vi "Get Ball.vi"() -> (0 "Field Relative X":dbl, 1 "Robot Relative Y":dbl, 3 "Robot Relative X":dbl, 4 "Ball Found?":bool)   [LabVIEW 2013]
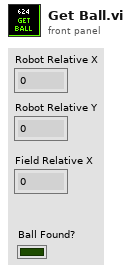
[diagram p1: front panel]
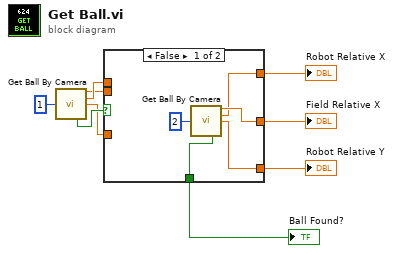
[diagram p0: block diagram]
diagram:
  n1 = call "Get Ball By Camera.vi"("Camera"=i16 1) -> ("Field Relative X"=w3:dbl, "Robot Relative X"=w7:dbl, "Robot Relative Y"=w5:dbl, "Ball Found?"=w8:bool)  [unwired: 9 in, 2 out]
  n2 = case shown="False" w8 {
    selector: w8 -> [_ w15]
    tunnel: w7 -> [_ w18]
    tunnel: [w10 w18] -> w6
    tunnel: w5 -> [_ w17]
    tunnel: [w12 w17] -> w4
    tunnel: w3 -> [_ w16]
    tunnel: [w11 w16] -> w2
    tunnel: [w13 w15] -> w1
    frame False {
      n3 = call "Get Ball By Camera.vi"("Camera"=i16 2) -> ("Field Relative X"=w11:dbl, "Robot Relative X"=w10:dbl, "Robot Relative Y"=w12:dbl, "Ball Found?"=w13:bool)  [unwired: 9 in, 2 out]
    }
    frame True {
    }
  }
  "Robot Relative X" <- w6
  "Field Relative X" <- w2
  "Robot Relative Y" <- w4
  "Ball Found?" <- w1
